vi "DeviceIsOpen.vi"(6 "Delay between send and receive [ms]":i32=100, 8 "error in (no error)":errorcluster, 11 "SCD in":refnum<class "SCD.lvclass">) -> (0 "error out":errorcluster, 1 "ID":i32, 2 "device is open?":bool, 3 "SCD out":refnum<class "SCD.lvclass">)   [LabVIEW 2023, in "horiba.lvlib" / "SCD.lvclass"]
doc: "Returns true if selected SpectrAcq3 is open."
uses:
  SCD.lvclass
  C:/Projects/Horiba/horiba-labview-sdk/Source/Classes/GenericDevice/GenericDevice.lvclass
  693ad44f-5526-43c4-bec2-cfa58c900c26.vi
  b95e9ea7-031b-4a20-81bd-e15d153e01c8.vi
  df1007d6-f737-4bfa-a2f6-95510aa9ddca.vi
  <vilib>/JDP Science/JSONtext/Find Item.vi
  <vilib>/JDP Science/JSONtext/Next JSON Value.vi
  <vilib>/JDP Science/JSONtext/String Subset.vi
  <vilib>/JDP Science/JSONtext/Parsing/Advance past next JSON Value (inlined COPY).vi
  <vilib>/JDP Science/JSONtext/Parsing/Advance past whitespace.vi
  <vilib>/JDP Science/JSONtext/Parsing/Advance past String.vi
  <vilib>/JDP Science/JSONtext/Parsing/Advance past Number.vi
  <vilib>/JDP Science/JSONtext/Parsing/Advance past Line Ending.vi
  <vilib>/JDP Science/JSONtext/Variant to JSON Text.vi
  <vilib>/JDP Science/JSONtext/Set Item.vi
  <vilib>/JDP Science/JSONtext/Parsing/Parse Full Path or Item Name.vi
  <vilib>/JDP Science/JSONtext/Parsing/Advance past Array.vi
  <vilib>/JDP Science/JSONtext/Parsing/Advance past Object.vi
  <vilib>/JDP Science/JSONtext/support/Error Cluster From Code.vi
  <vilib>/JDP Science/JSONtext/Offset/Find Item Locations by Path.vi
  <vilib>/JDP Science/JSONtext/JSON text to Variant.vi
  <vilib>/JDP Science/JSONtext/LVClass Serializer/JSONtext LVClass Serializer.lvclass
  SCD.lvclass/SCD.ctl
  GenericDevice/GenericDevice.lvclass
panel:
  out "Found":bool
  # "Connector Pane"
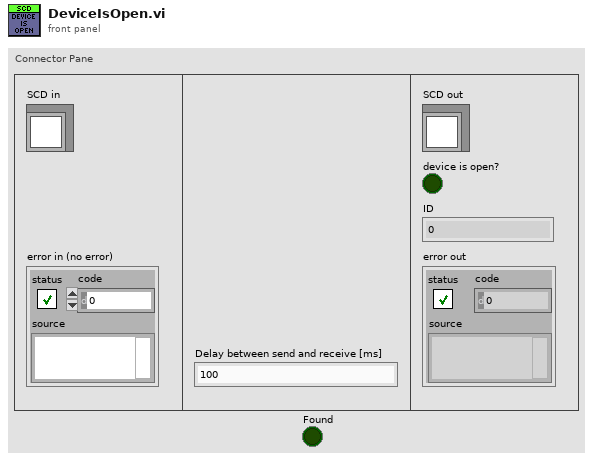
[diagram p1: front panel]
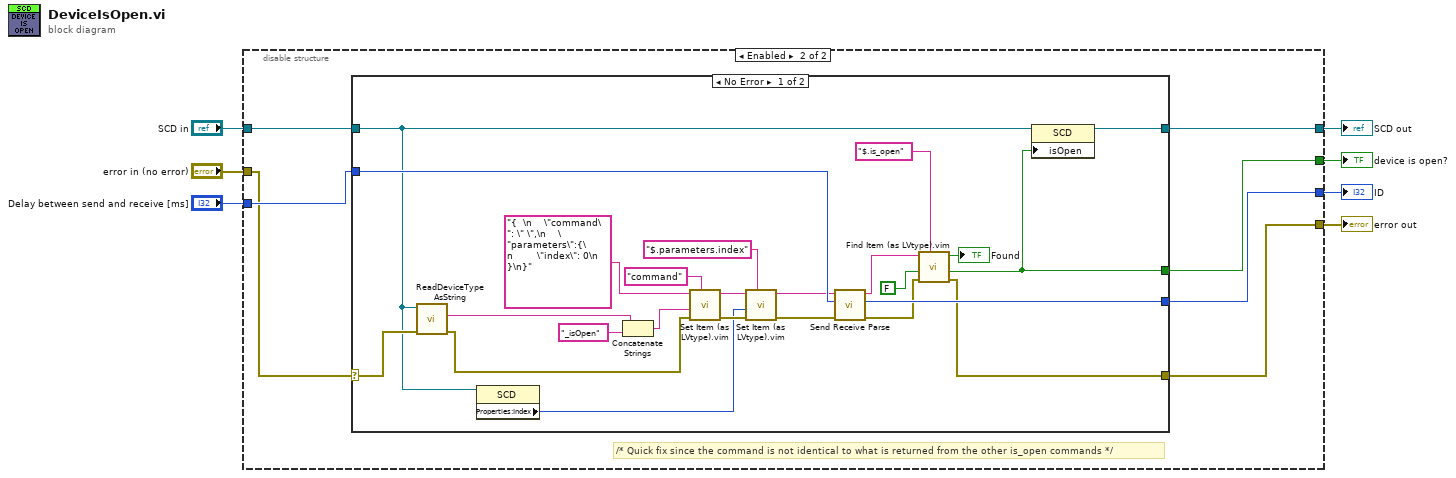
[diagram p0: block diagram]
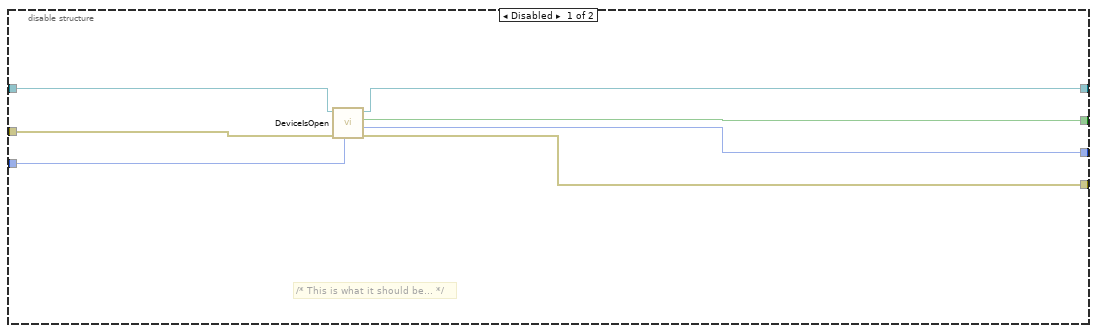
[diagram p2: hidden frame]
diagram:
  n1 = disable-structure shown="Enabled" {
    disable-tunnel: [w14 w18] -> w7
    disable-tunnel: [w13 w15] -> w6
    disable-tunnel: [w12 w16] -> w5
    disable-tunnel: [w11 w17] -> w4
    disable-tunnel: "error in (no error)" -> [w10 w19]
    disable-tunnel: "SCD in" -> [w9 w21]
    disable-tunnel: "Delay between send and receive [ms]" -> [w8 w20]
    frame Disabled {
      # "/* This is what it should be... */"
      n2 = call-parent "DeviceIsOpen.vi"("Delay between send and receive [ms]"=w8, "error in (no error)"=w10, "GenericDevice in"=w9) -> ("error out"=w14:errorcluster, "ID"=w13:i32, "device is open?"=w12:bool, "GenericDevice out"=w11:refnum<class "SCD.lvclass">)  [unwired: 5 in]
    }
    frame Enabled {
      # "/* Quick fix since the command is not identical to what is returned from the other is_open commands */"
      n3 = case shown="No Error" w19 {
        selector: w19 -> [w36 w47]
        tunnel: [w23 w47] -> w18
        tunnel: [w31 w46] -> w17
        tunnel: w21 -> [w26 w46]
        tunnel: [w28 _] -> w16
        tunnel: [w37 _] -> w15
        tunnel: w20 -> [w33 _]
        frame No Error {
          n4 = call "ReadDeviceTypeAsString.vi"("error in (no error)"=w36, "GenericDevice In"=w26) -> ("error out"=w35:errorcluster, "String"=w34:string)  [unwired: 7 in, 1 out]
          n5 = property class="SCD"(reference=w26) -> ("Properties:Index"=w25:i32)  [unwired: 1 in, 2 out]
          n6 = Concatenate Strings(w34, "_isOpen" ("string")) -> (w39:string)
          n7 = call "Set Item (as LVtype).vim"("$Path or Item Name"="command", "error in (no error)"=w35, "Anything"=w39, "JSON"="{  \n    \"command\": \" \",\n    \"parameters\":{\n        \"index\": 0\n    }\n}") -> ("error out"=w43:errorcluster, "<JSON>"=w44:string)  [unwired: 4 in, 1 out]
          n8 = call "Set Item (as LVtype).vim"("$Path or Item Name"="$.parameters.index", "error in (no error)"=w43, "Anything"=w25, "JSON"=w44) -> ("error out"=w38:errorcluster, "<JSON>"=w32:string)  [unwired: 4 in, 1 out]
          n9 = call "Send Receive Parse.vi"("error in"=w38, "Delay between send and receive [ms]"=w33, "<JSON>"=w32) -> ("error out"=w24:errorcluster, "ID"=w37:i32, "results-JSON string"=w30:string)  [unwired: 6 in]
          n10 = call "Find Item (as LVtype).vim"("$Path or Item Name"="$.is_open", "error in (no error)"=w24, "Data Type and Default Value"=FALSE, "JSON"=w30) -> ("error out"=w23:errorcluster, "Data"=w28:bool, "Found"=→"Found":bool)  [unwired: 4 in, 1 out]
          n11 = property class="SCD"(reference=w26, "isOpen"=w28) -> (reference out=w31:refnum<class "SCD.lvclass">)  [unwired: 1 in, 1 out]
        }
        frame Error {
        }
      }
    }
  }
  "error out" <- w7
  "SCD out" <- w4
  "ID" <- w6
  "device is open?" <- w5
